vi "QueryIdentification.vi"(1 "Destination":T1={"Subsystem Id"=90, "Node Id"=1, "Component Id"=1}, 3 "QueryType":u8=2, 4 "Source":T1={"Subsystem Id"=3, "Node Id"=1, "Component Id"=1}) -> (0 "Encoded JAUS Message":string)   [LabVIEW 2011]
uses:
  Support Files/Address.ctl
panel:
  in  "Command Code":string="+\u0000"
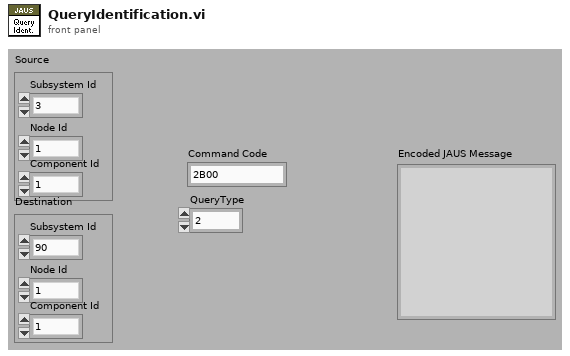
[diagram p1: front panel]
types:
  T1 = typedef "Address.ctl" = cluster{"Subsystem Id":u16, "Node Id":u8, "Component Id":u8}
  T2 = cluster{"unsigned byte array[0]":u8, "unsigned byte array[1]":u8}
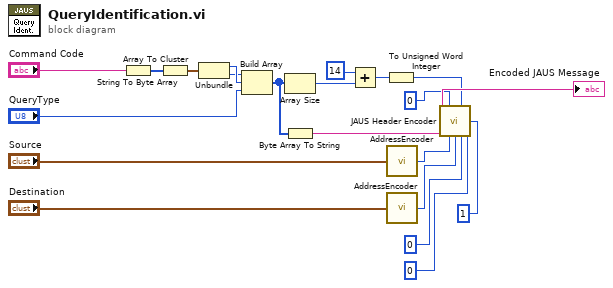
[diagram p0: block diagram]
diagram:
  n1 = String To Byte Array(string="Command Code") -> (unsigned byte array=w7:u8[])
  n2 = Array To Cluster(array=w7) -> (cluster=w6:T2)
  n3 = Unbundle(w6) -> ("unsigned byte array[0]"=w5:u8, "unsigned byte array[1]"=w4:u8)
  n4 = Build Array(w4, w5, "QueryType") -> (w11:u8[])
  n5 = Array Size(array=w11) -> (size(s)=w9:i32)
  n6 = Byte Array To String(unsigned byte array=w11) -> (string=w13:string)
  n7 = Add(x=14, y=w9) -> (x+y=w8:i32)
  n8 = To Unsigned Word Integer(number=w8) -> (unsigned 16bit integer=w1:u16)
  n9 = call "AddressEncoder.vi"("Address Cluster"="Source") -> ("Address"=w20:u32)
  n10 = call "AddressEncoder.vi"("Address Cluster"="Destination") -> ("Address"=w19:u32)
  n11 = call "JAUS Header Encoder.vi"("Message Type (0-5)"=u8 0, "Data Size (8-23)"=w1, "Priority(40-41)"=u8 1, "Payload"=w13, "Source ID (80-95)"=w20, "Destination ID (48-79)"=w19, "Data Flags (46-47)"=u8 0, "Ack/Nak (44-45)"=u8 0) -> ("Encoded JAUS Message"=→"Encoded JAUS Message":string)  [unwired: 7 in]
